vi "small_Desktop Main.vi"() -> ()   [LabVIEW 2018]
doc: "Demonstrates the use of the Network Streams functions to send LED status to the myRIO target."
uses:
  <vilib>/ErrorRing/Error Ring.xnode
panel:
  in  "Pause":bool
  out "Array":dbl[](array[numeric])
  in  "Parameter Settings":T1(tab)=enum."Conical Field" caption="Field Types"
  in  "fg":dbl
  in  "pg":dbl
  in  "dg":dbl
  in  "Ag":dbl
  in  "AoOF":dbl
  in  "fo":sgl
  in  "do":sgl
  in  "oo":sgl
  in  "po":sgl
  in  "cc":sgl
  in  "pc":sgl
  in  "wc":sgl
  in  "dc":sgl
  in  "Ac":dbl
  in  "pr":sgl
  in  "Ar":dbl
  in  "wr":sgl
  in  "dr":sgl
  in  "Dis phase step":dbl
  in  "Dis phase frequency (Hz)":dbl
  in  "Dis tumbling frequency (Hz)":dbl
  in  "Dis strength(mT)":dbl
  in  "Swa strength (mT)":dbl
  in  "Swa frequency (Hz)":dbl
  in  "Swa pitch angle (deg)":dbl
  in  "Swa direction angle (deg)":dbl
  in  "Swa ratio":dbl=1.0
  in  "Pitch Angle (rotating around Constant, deg)":dbl
  in  "Ratio (A/C)":sgl
  in  "Direction Angle (deg)":sgl
  in  "Pitch Angle (rotating around Origin, deg)":sgl
  in  "Frequency (Hz)":sgl
  in  "Strength (mT)":dbl
  in  "Ar 2":dbl caption="Ar"
  in  "ratio":sgl
  in  "pr  2":sgl
  in  "dr  2":sgl
  in  "wr  2":sgl
  in  "p_x":sgl
  out "Numeric 5":i32
  in  "Stop":bool
  out "error out":errorcluster
  in  "Target IP Address":string="172.22.11.2"
  # "Overview: Magnetic field calculation, and send parameters to myRIO\nInstructions:\n1. Verify the value of Target IP Address. Set Visa resource name.\n2. Ensure RT Main.vi is already running. \n3. Run this VI. Set parameters of magnetic field."
  # "Strength (mT)"
  # "Pitch Angle (deg)"
  # "Direction Angle (deg)"
  # "Frequency (Hz)"
  # "Strength (mT)"
  # "Oscilation Frequency (Hz)"
  # "Oscilation Angle (deg)"
  # "Pitch Angle (deg)"
  # "Direction Angle (deg)"
  # "Strength (mT)"
  # "Frequency (Hz)"
  # "Pitch Angle (deg)"
  # "Direction Angle (deg)"
  # "Conical Angle (deg)"
  # "Strength (mT)"
  # "Frequency (Hz)"
  # "Pitch Angle (deg)"
  # "Direction Angle (deg)"
  # "Strength (mT)"
  # "Tumbling Frequency (Hz)"
  # "Phase Frequency (Hz)"
  # "Phase Step"
  # "Strength (mT)"
  # "Frequency (Hz)"
  # "Pitch Angle (deg)"
  # "Direction Angle (deg)"
  # "Ratio"
  # "Strength (mT)"
  # "Frequency (Hz)"
  # "Ratio (A/C)"
  # "Direction Angle (deg)"
  # "Pitch Angle (rotating around Origin, deg)"
  # "Pitch Angle (rotating around Constant, deg)"
  # "Strength (mT)"
  # "Frequency (Hz)"
  # "Pitch Angle Y (deg)"
  # "Pitch Angle X (deg)"
  # "Direction Angle (deg)"
  # "ratio (l/s)"
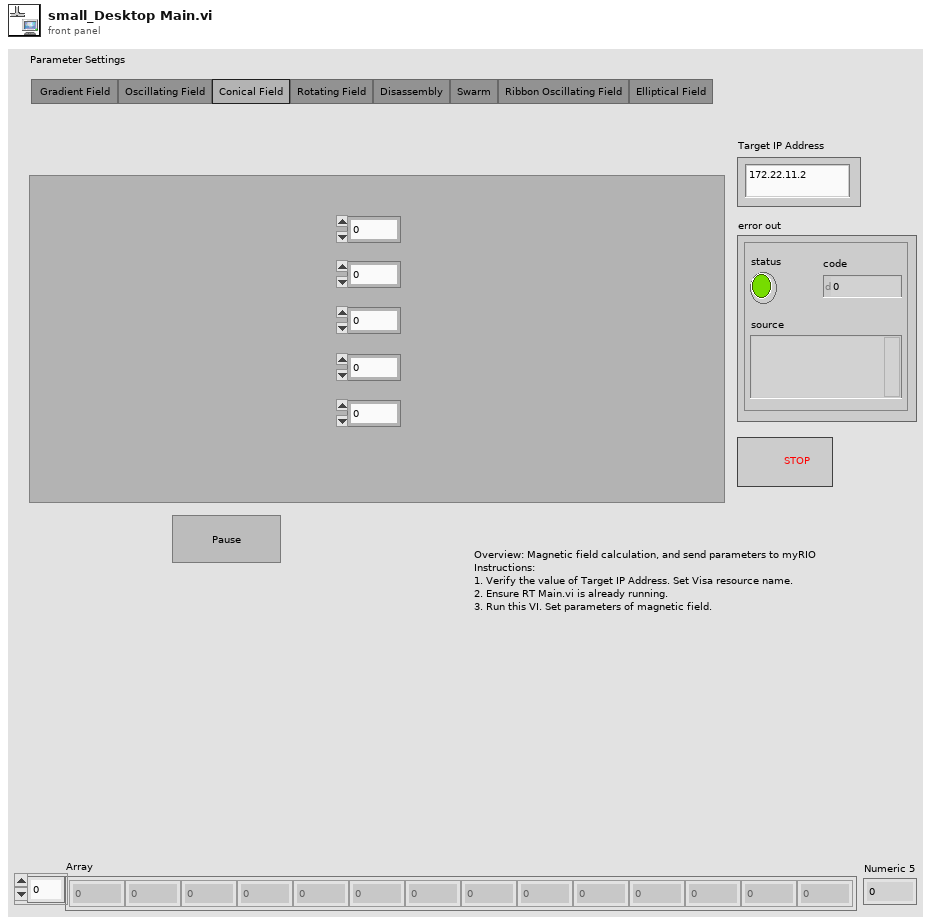
[diagram p1: front panel]
types:
  T1 = enum32{"Gradient Field ", "Oscillating Field", "Conical Field", "Rotating Field", "Disassembly", "Swarm", "Ribbon Oscillating Field", "Elliptical Field"}
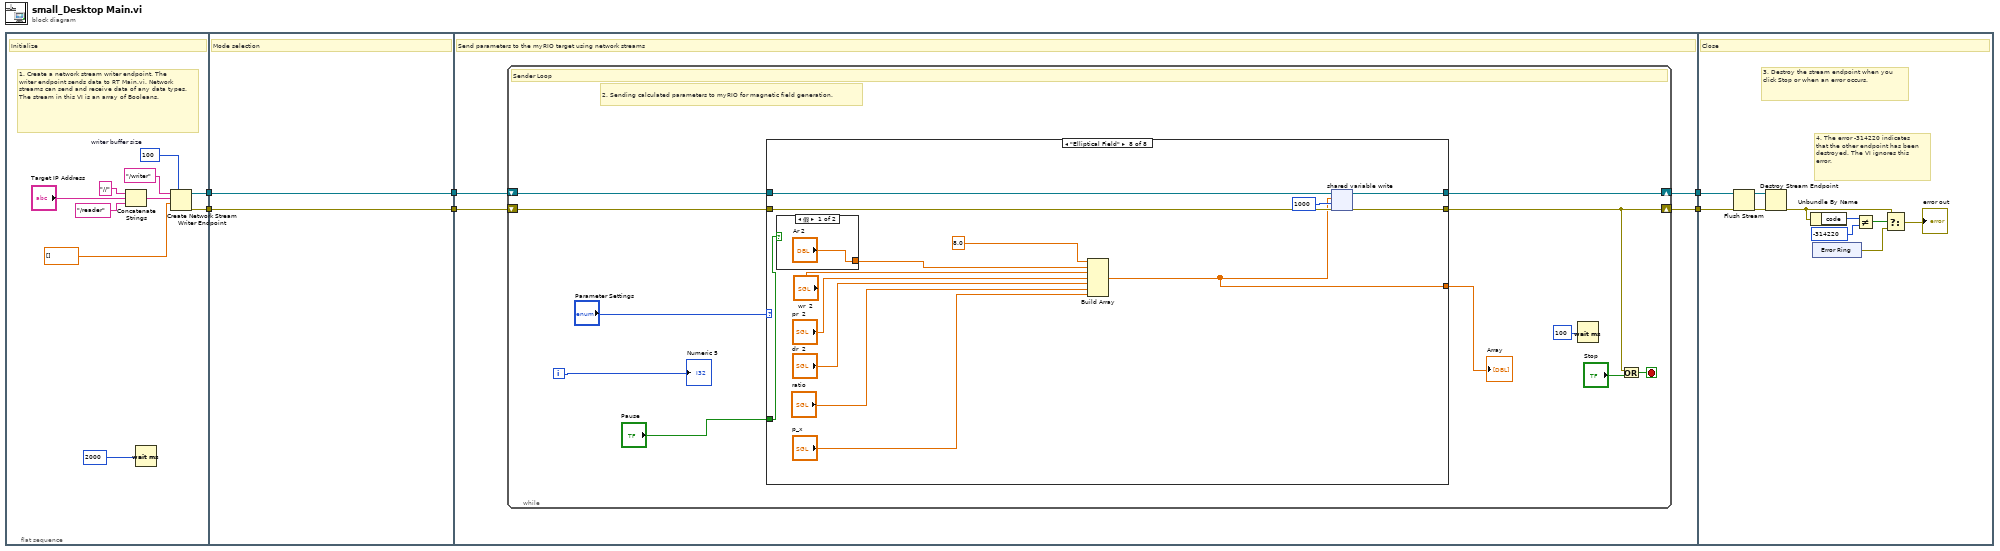
[diagram p0: block diagram]
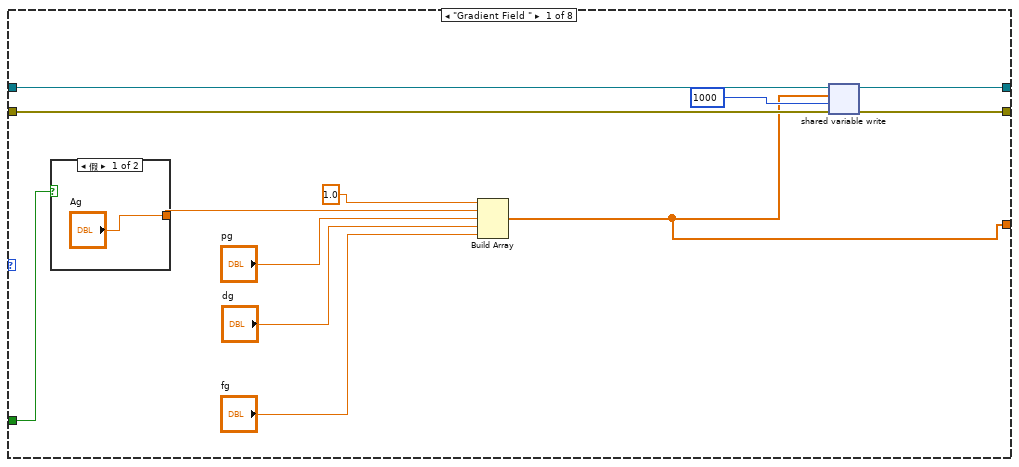
[diagram p2: hidden frame]
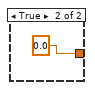
[diagram p3: hidden frame]
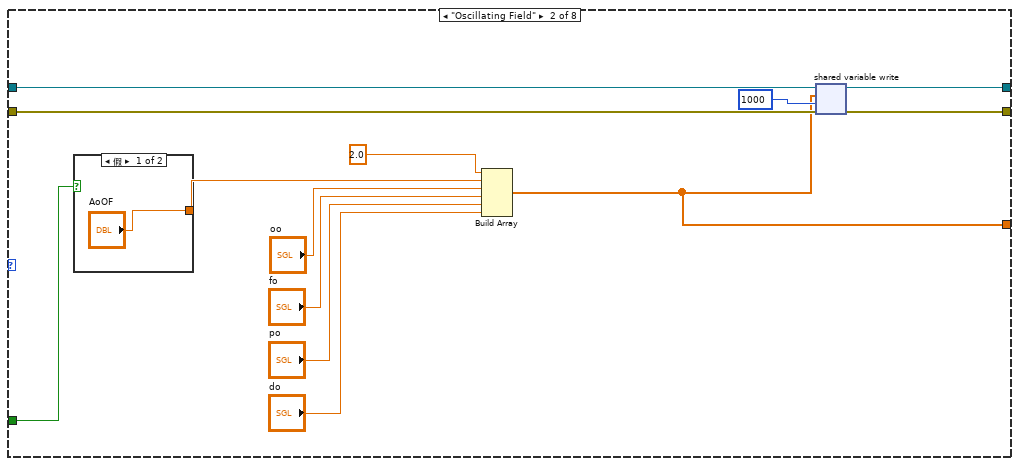
[diagram p4: hidden frame]
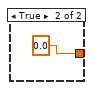
[diagram p5: hidden frame]
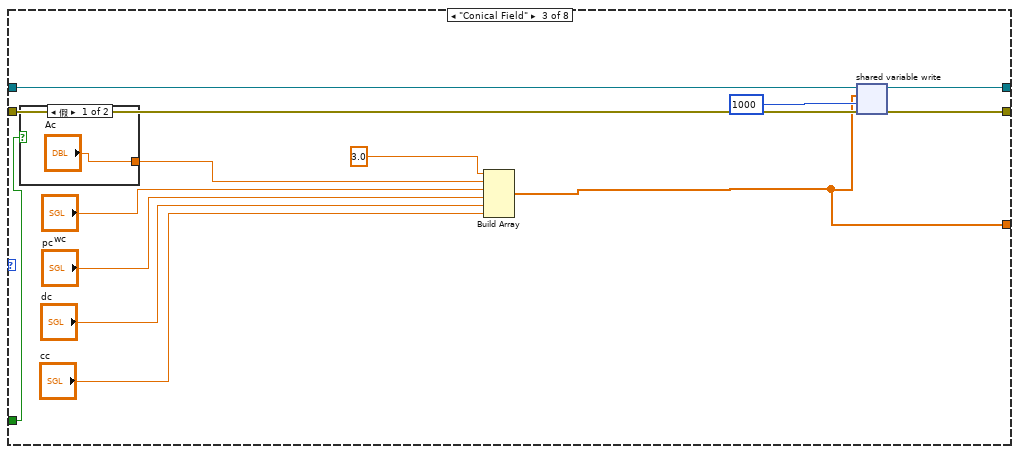
[diagram p6: hidden frame]
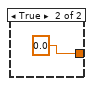
[diagram p7: hidden frame]
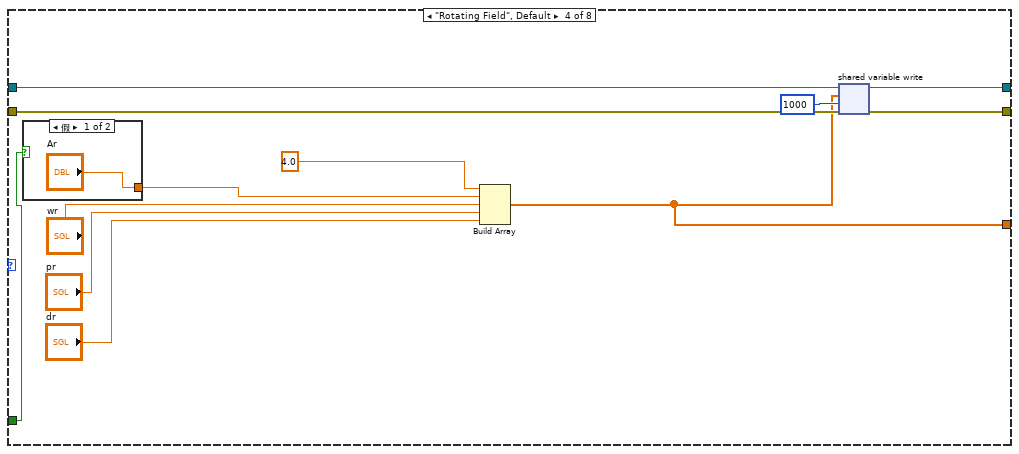
[diagram p8: hidden frame]
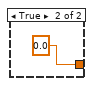
[diagram p9: hidden frame]
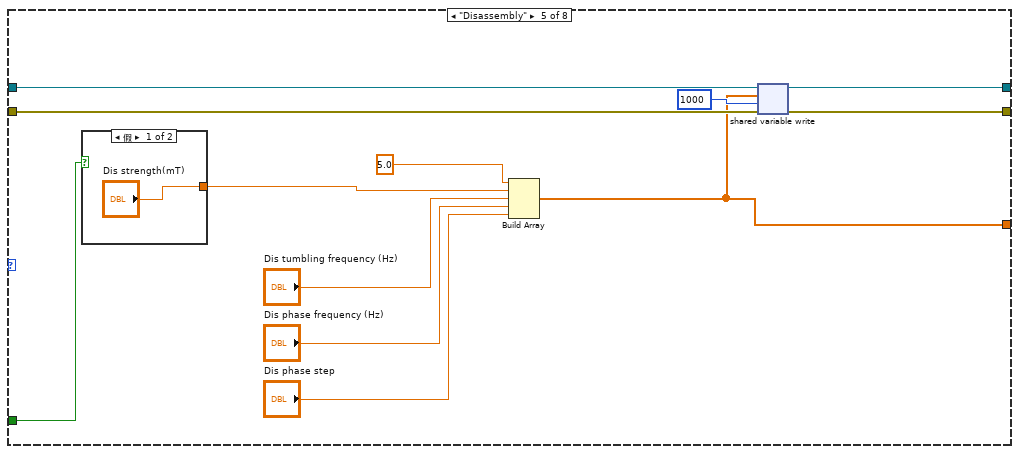
[diagram p10: hidden frame]
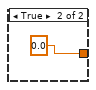
[diagram p11: hidden frame]
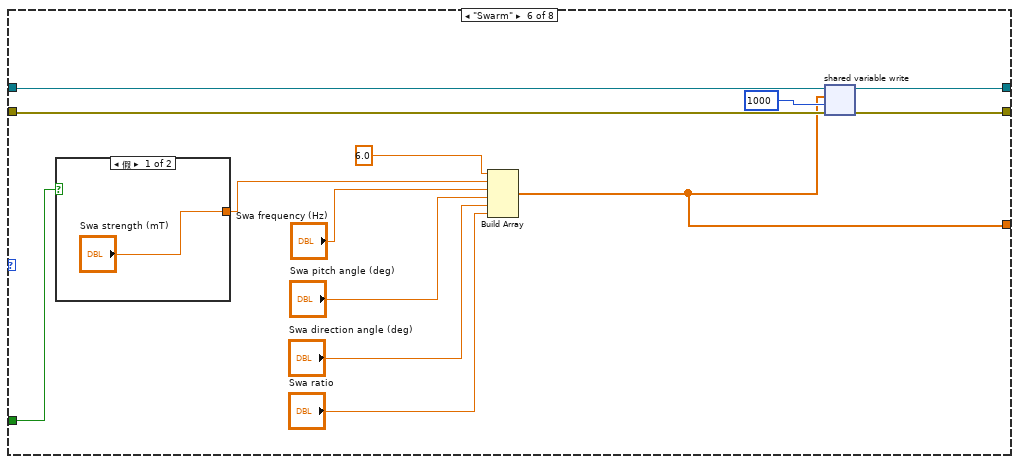
[diagram p12: hidden frame]
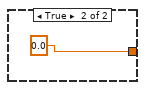
[diagram p13: hidden frame]
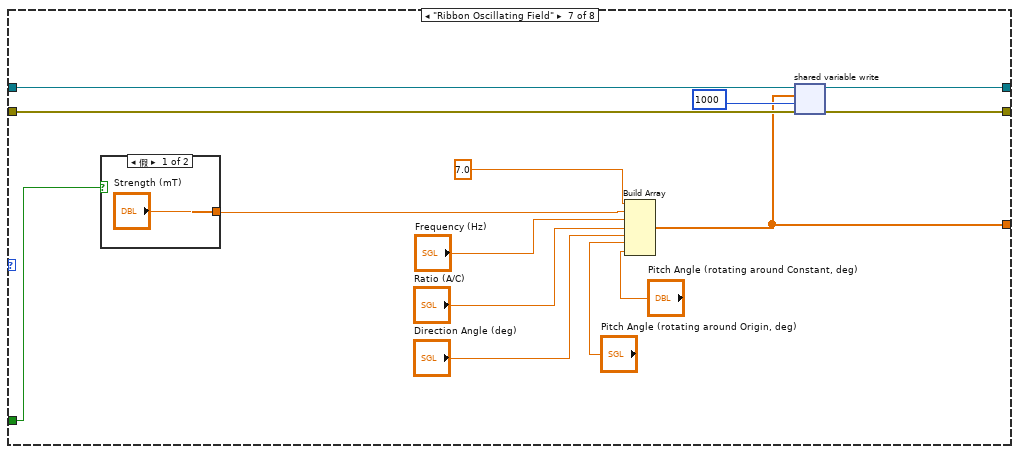
[diagram p14: hidden frame]
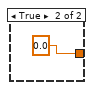
[diagram p15: hidden frame]
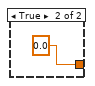
[diagram p16: hidden frame]
diagram:
  n1 = flat-sequence {
    tunnel: [w11] -> w2
    tunnel: [w10] -> w1
    tunnel: [w18] -> w4
    tunnel: [w17] -> w3
    tunnel: w1 -> [w17]
    tunnel: w2 -> [w18]
    tunnel: [w20] -> w6
    tunnel: w4 -> [w22]
    tunnel: [w19] -> w5
    tunnel: w3 -> [w21]
    tunnel: w6 -> [w162]
    tunnel: w5 -> [w159]
    frame #0 {
      w9 = 100  # writer buffer size
      # "1. Create a network stream writer endpoint. The writer endpoint sends data to RT Main.vi. Network streams can send and receive data of any data types. The stream in this VI is an array of Booleans."
      # "Initialize"
      n2 = Concatenate Strings("//", "Target IP Address", "/reader") -> (w16:string)
      n3 = Wait (ms)(milliseconds to wait=2000) -> ()  [unwired: 1 out]
      n4 = Create Network Stream Writer Endpoint(7:w9, 9:dbl[] [], 10:w16, 11:"/writer" ("reader name")) -> (0:w10:errorcluster, 3:w11:refnum<k21>)  [unwired: 3 in]
    }
    frame #1 {
      # "Mode selection"
    }
    frame #2 {
      # "Send parameters to the myRIO target using network streams"
      n5 = while {
        shift-right: [w26] -> w19
        shift-left: w21 -> [w28]
        shift-right: [w27] -> w20
        shift-left: w22 -> [w29]
        i -> [w30]
        stop <- w33 stop-if-true
        # "2. Sending calculated parameters to myRIO for magnetic field generation."
        # "Sender Loop"
        n6 = case shown="\"Elliptical Field\"" "Parameter Settings" {
          tunnel: w29 -> [w44 w59 w74 w88 w102 w116 w134 w149]
          tunnel: w28 -> [w41 w58 w73 w87 w100 w115 w132 w148]
          tunnel: [w43 w57 w71 w86 w101 w114 w133 w147] -> w27
          tunnel: [w42 w56 w72 w85 w99 w113 w131 w146] -> w26
          tunnel: [w37 w50 w65 w80 w93 w108 w129 w141] -> w25
          tunnel: "Pause" -> [w35 w48 w63 w78 w92 w107 w124 w139]
          frame "Gradient Field " {
            n7 = case shown="假" w35 {
              tunnel: ["Ag" 0.0] -> w36
              frame False {
              }
              frame True {
              }
            }
            n8 = Build Array(1.0, w36, "pg", "dg", "fg") -> (w37:dbl[])
            n9 = shared-variable-write(w44, w41, w37, 1000 ("timeout ms (-1)")) -> (w43:refnum<k21>, w42:errorcluster)  [unwired: 1 out]
          }
          frame "Oscillating Field" {
            n10 = case shown="假" w48 {
              tunnel: ["AoOF" 0.0] -> w49
              frame False {
              }
              frame True {
              }
            }
            n11 = Build Array(2.0, w49, "oo", "fo", "po", "do") -> (w50:dbl[])
            n12 = shared-variable-write(w59, w58, w50, 1000 ("timeout ms (-1)")) -> (w57:refnum<k21>, w56:errorcluster)  [unwired: 1 out]
          }
          frame "Conical Field" {
            # "FG"
            n13 = case shown="假" w63 {
              tunnel: ["Ac" 0.0] -> w64
              frame False {
              }
              frame True {
              }
            }
            n14 = Build Array(3.0, w64, "wc", "pc", "dc", "cc") -> (w65:dbl[])
            n15 = shared-variable-write(w74, w73, w65, 1000 ("timeout ms (-1)")) -> (w71:refnum<k21>, w72:errorcluster)  [unwired: 1 out]
          }
          frame "Rotating Field", Default {
            n16 = case shown="假" w78 {
              tunnel: ["Ar" 0.0] -> w79
              frame False {
              }
              frame True {
              }
            }
            n17 = Build Array(4.0, w79, "wr", "pr", "dr") -> (w80:dbl[])
            n18 = shared-variable-write(w88, w87, w80, 1000 ("timeout ms (-1)")) -> (w86:refnum<k21>, w85:errorcluster)  [unwired: 1 out]
          }
          frame "Disassembly" {
            n19 = case shown="假" w92 {
              tunnel: ["Dis strength(mT)" 0.0] -> w97
              frame False {
              }
              frame True {
              }
            }
            n20 = Build Array(5.0, w97, "Dis tumbling frequency (Hz)", "Dis phase frequency (Hz)", "Dis phase step") -> (w93:dbl[])
            n21 = shared-variable-write(w102, w100, w93, 1000 ("timeout ms (-1)")) -> (w101:refnum<k21>, w99:errorcluster)  [unwired: 1 out]
          }
          frame "Swarm" {
            n22 = case shown="假" w107 {
              tunnel: ["Swa strength (mT)" 0.0] -> w106
              frame False {
              }
              frame True {
              }
            }
            n23 = Build Array(6.0, w106, "Swa frequency (Hz)", "Swa pitch angle (deg)", "Swa direction angle (deg)", "Swa ratio") -> (w108:dbl[])
            n24 = shared-variable-write(w116, w115, w108, 1000 ("timeout ms (-1)")) -> (w114:refnum<k21>, w113:errorcluster)  [unwired: 1 out]
          }
          frame "Ribbon Oscillating Field" {
            n25 = case shown="假" w124 {
              tunnel: ["Strength (mT)" 0.0] -> w123
              frame False {
              }
              frame True {
              }
            }
            n26 = Build Array(7.0, w123, "Frequency (Hz)", "Ratio (A/C)", "Direction Angle (deg)", "Pitch Angle (rotating around Origin, deg)", "Pitch Angle (rotating around Constant, deg)") -> (w129:dbl[])
            n27 = shared-variable-write(w134, w132, w129, 1000 ("timeout ms (-1)")) -> (w133:refnum<k21>, w131:errorcluster)  [unwired: 1 out]
          }
          frame "Elliptical Field" {
            n28 = case shown="假" w139 {
              tunnel: ["Ar 2" 0.0] -> w140
              frame False {
              }
              frame True {
              }
            }
            n29 = Build Array(8.0, w140, "wr  2", "pr  2", "dr  2", "ratio", "p_x") -> (w141:dbl[])
            n30 = shared-variable-write(w149, w148, w141, 1000 ("timeout ms (-1)")) -> (w147:refnum<k21>, w146:errorcluster)  [unwired: 1 out]
          }
        }
        "Array" <- w25
        n31 = Wait (ms)(milliseconds to wait=u32 100) -> ()  [unwired: 1 out]
        n32 = Or(x=w26, y="Stop") -> (x .or. y?=w33:bool)
        "Numeric 5" <- w30
      }
    }
    frame #3 {
      # "4. The error -314220 indicates that the other endpoint has been destroyed. The VI ignores this error."
      # "3. Destroy the stream endpoint when you click Stop or when an error occurs."
      # "Close"
      n33 = Flush Stream(8:w159, 11:w162) -> (0:w160:errorcluster, 3:w161:refnum<k21>)  [unwired: 2 in, 1 out]
      n34 = Destroy Stream Endpoint(8:w160, 11:w161) -> (0:w154:errorcluster)
      n35 = Unbundle By Name(w154) -> ("code"=w158:i32)
      n36 = xnode "Error Ring"() -> ("错误输出"=w155:errorcluster)
      n37 = Not Equal?(x=w158, y=-314220) -> (x != y?=w156:bool)
      n38 = Select(t=w154, s=w156, f=w155) -> (s? t:f=→"error out":errorcluster)
    }
  }
